vi "Determine Warnings.vi"(8 "에러 입력(에러 없음)":errorcluster, 9 "최저 온도":dbl, 10 "최고 온도":dbl, 11 "현재 온도":dbl) -> (0 "에러 출력":errorcluster, 1 "경고?":bool, 2 "경고 텍스트":string)   [LabVIEW 2010]
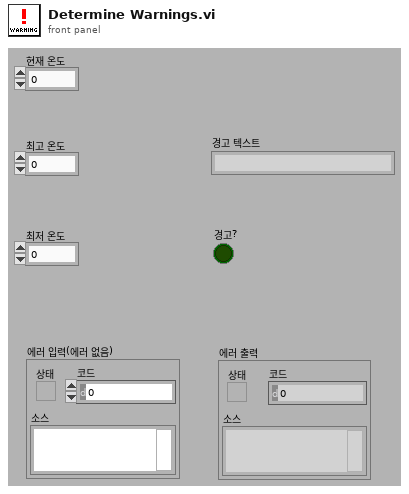
[diagram p1: front panel]
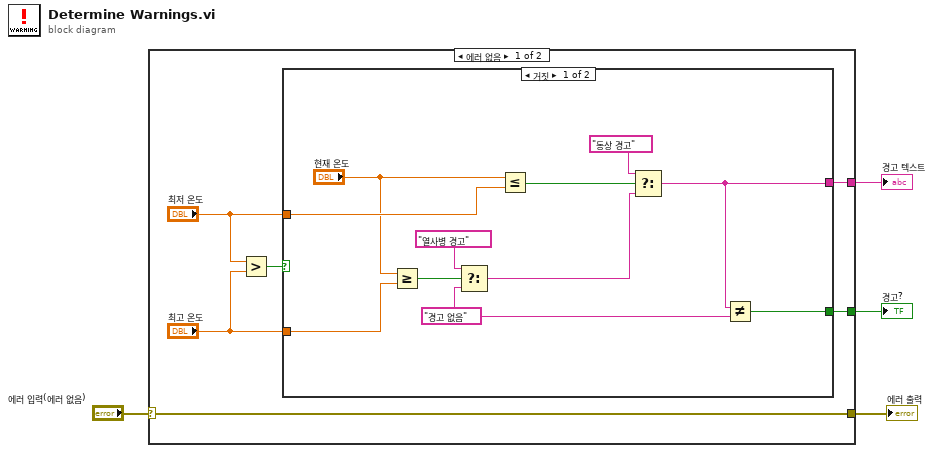
[diagram p0: block diagram]
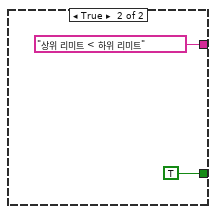
[diagram p2: hidden frame]
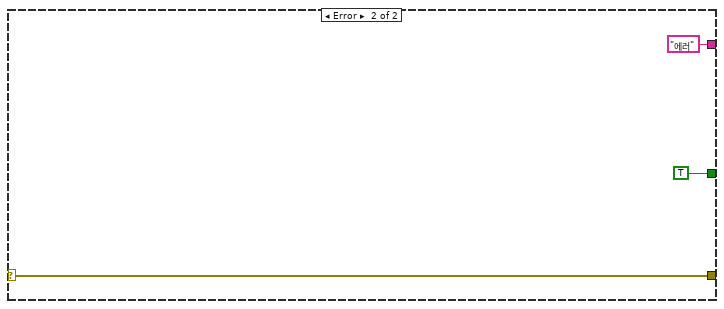
[diagram p3: hidden frame]
diagram:
  n1 = case shown="에러 없음" "에러 입력(에러 없음)" {
    selector: "에러 입력(에러 없음)" -> [w5 w26]
    tunnel: [w10 "에러" ("f")] -> w4
    tunnel: [w9 TRUE] -> w3
    tunnel: [w5 w26] -> w1
    frame No Error {
      n2 = Greater?(x="최저 온도", y="최고 온도") -> (0:w8:bool)
      n3 = case shown="거짓" w8 {
        tunnel: [w21 "상위 리미트 < 하위 리미트" ("f")] -> w10
        tunnel: [w20 TRUE] -> w9
        tunnel: "최고 온도" -> [w19 _]
        tunnel: "최저 온도" -> [w16 _]
        frame False {
          w11 = "경고 없음" ("f")
          n4 = Greater Or Equal?(x="현재 온도", y=w19) -> (x >= y?=w18:bool)
          n5 = Select(t="열사병 경고", s=w18, f=w11) -> (s? t:f=w12:string)
          n6 = Less Or Equal?(x="현재 온도", y=w16) -> (x <= y?=w13:bool)
          n7 = Select(t="동상 경고", s=w13, f=w12) -> (s? t:f=w21:string)
          n8 = Not Equal?(x=w21, y=w11) -> (x != y?=w20:bool)
        }
        frame True {
        }
      }
    }
    frame Error {
    }
  }
  "경고 텍스트" <- w4
  "경고?" <- w3
  "에러 출력" <- w1
